vi "Sefram DAS220 - Configure start trigger and Record.vi"() -> ()   [LabVIEW 2017, in "Sefram DAS220.lvlib"]
doc: "Configure an analog channel and start trigger to start recording."
uses:
  <instrlib>/Sefram DAS220/Sefram DAS220.lvlib
  <instrlib>/Sefram DAS220/Public/Configure/Triggers-Alarms/Low-level/Trigger Types/Complex Trigger Consign.ctl
  <instrlib>/Sefram DAS220/Public/Configure/Channels/Low-level/Set Type Voltage.vi
  <instrlib>/Sefram DAS220/Public/Configure/Triggers-Alarms/Low-level/Start Trigger/Start Trigger Simple Analog Channel.vi
panel:
  in  "Trigger consign":T1 {"Channel" items=["A1"=0, "A2"=1, "A3"=2, "A4"=3, "A5"=4, "A6"=5, "A7"=6, "A8"=7, "A9"=8, "A10"=9, "K1"=200, "K2"=201, "K3"=202, "K4"=203, "FA1"=204, "FA2"=205, "FA3"=206, "FA4"=207]; "Assign to S1 or S2 threshold?" items=["S1", "S2"]; "Positive or negative (edge or level)" items=["Positive", "Negative"]}
  in  "Channel":u16(ring) items=["A1"=0, "A2"=1, "A3"=2, "A4"=3, "A5"=4, "A6"=5, "A7"=6, "A8"=7, "A9"=8, "A10"=9, "K1"=200, "K2"=201, "K3"=202, "K4"=203, "FA1"=204, "FA2"=205, "FA3"=206, "FA4"=207]
  in  "Sampling Period":u16(ring)=10 items=["1ms"=1, "2ms"=2, "5ms"=5, "10ms"=10, "20ms"=20, "50ms"=50, "100ms"=100]
  in  "VISA resource name":refnum<visa-resource-name>
  # "Channel Settings"
  # "Configure selected channel as voltage input, sampling period at 10ms.\nStart trigger is set at 2,65V, so recording will start when voltage will reach that value.\n\nThen record will start and wait for trigger."
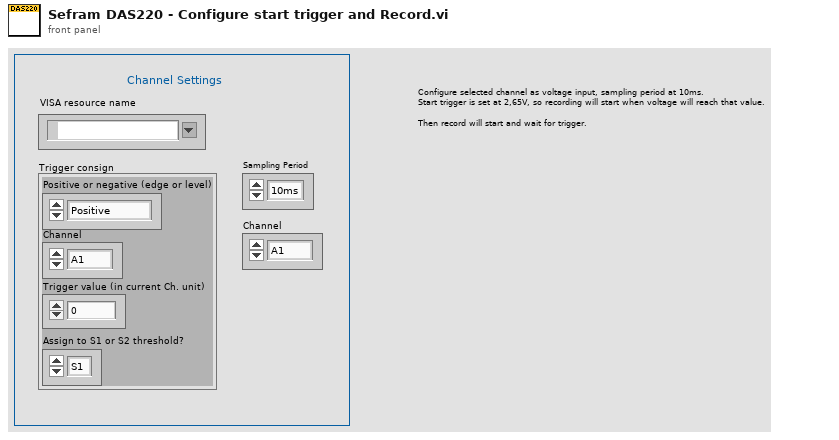
[diagram p1: front panel]
types:
  T1 = typedef "Sefram DAS220.lvlib/Complex Trigger Consign.ctl" = cluster{"Trigger value (in current Ch. unit)":dbl, "Positive or negative (edge or level)":u16, "Assign to S1 or S2 threshold?":u16, "Channel":u16}
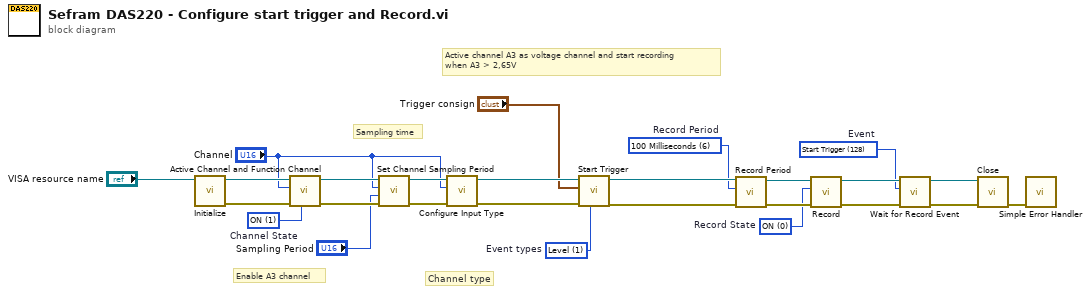
[diagram p0: block diagram]
diagram:
  w4 = u16 128 items=["Record Start"=32, "Record End"=64, "Start Trigger"=128]  # Event
  w9 = u16 0 items=["ON", "OFF", "TRIG"]  # Record State
  w12 = u16 1 items=["Edge", "Level"]  # Event types
  w14 = u16 6 items=["1 Millisecond", "2 Milliseconds", "5 Milliseconds", "10 Milliseconds", "20 Milliseconds", "50 Milliseconds", "100 Milliseconds", "200 Milliseconds", "500 Milliseconds", "1 Second", "2 Seconds", "5 Seconds", "10 Seconds", "20 Seconds", "1 Minute", "2 Minutes", "5 Minutes", "10 Minutes", "20 Minutes"]  # Record Period
  w20 = u16 1 items=["OFF", "ON"]  # Channel State
  # "Active channel A3 as voltage channel and start recording\nwhen A3 > 2,65V"
  # "Sampling time"
  # "Channel type"
  # "Enable A3 channel"
  n1 = call <instrlib>:"Initialize.vi"("VISA resource name"="VISA resource name") -> ("error out"=w25:errorcluster, "VISA resource name out"=w26:refnum<visa-resource-name>)  [unwired: 9 in]
  n2 = call <instrlib>:"Active Channel and Function Channel.vi"("Channel State"=w20, "error in (no error)"=w25, "Channel"="Channel", "VISA resource name"=w26) -> ("error out"=w23:errorcluster, "VISA resource name out"=w22:refnum<visa-resource-name>)  [unwired: 6 in]
  n3 = call <instrlib>:"Set Channel Sampling Period.vi"("error in (no error)"=w23, "Sampling Period"="Sampling Period", "Channel"="Channel", "VISA resource name"=w22) -> ("error out"=w24:errorcluster, "VISA resource name out"=w21:refnum<visa-resource-name>)  [unwired: 6 in]
  n4 = call-poly <instrlib>:"Configure Input Type.vi"("error in (no error)"=w24, "Channel"="Channel", "VISA resource name"=w21) -> ("error out"=w17:errorcluster, "VISA resource name out"=w18:refnum<visa-resource-name>)  [unwired: 7 in]
  n5 = call-poly <instrlib>:"Start Trigger.vi"("Event types (Edge or Level)"=w12, "error in (no error)"=w17, "Trigger consign"="Trigger consign", "VISA resource name"=w18) -> ("error out"=w15:errorcluster, "VISA resource name out"=w16:refnum<visa-resource-name>)  [unwired: 6 in]
  n6 = call <instrlib>:"Record Period.vi"("error in (no error)"=w15, "Record Period"=w14, "VISA resource name"=w16) -> ("error out"=w10:errorcluster, "VISA resource name out"=w11:refnum<visa-resource-name>)  [unwired: 7 in]
  n7 = call <instrlib>:"Record.vi"("error in (no error)"=w10, "Record State"=w9, "VISA resource name"=w11) -> ("error out"=w7:errorcluster, "VISA resource name out"=w8:refnum<visa-resource-name>)  [unwired: 7 in]
  n8 = call <instrlib>:"Wait for Record Event.vi"("error in"=w7, "Event"=w4, "VISA resource name"=w8) -> ("error out"=w5:errorcluster, "VISA resource name out"=w6:refnum<visa-resource-name>)  [unwired: 7 in]
  n9 = call <instrlib>:"Close.vi"("error in (no error)"=w5, "VISA resource name"=w6) -> ("error out"=w1:errorcluster)  [unwired: 9 in]
  n10 = call <vilib>:"Simple Error Handler.vi"("error in (no error)"=w1) -> ()  [unwired: 4 in, 5 out]
